vi "importAcq.vi"(7 "Probes":enum16{"Testing", "1-5", "6-10"}(ring)=enum."6-10", 8 "error in (no error)":errorcluster, 9 "Params":T1={"Mice ID"=[], "ExpType"=[], "Trial Interval"=[], "Pulse Duration"=[158.0, 152.0, 156.0, 167.0, 172.0], "microL_per_pulse"=[6.0, 6.0, 6.0, 6.0, 6.0], "Response Interval"=[1000.0, 1000.0, 1000.0, 1000.0, 1000.0], "Bad Delay"=[], "Response Period"=[], "liquid_type"="water", "Stimuli"=[], "Rewarded Stimuli"=[], "Air Dur"=50.0} {"Air Dur" format="%#_13g"}, 10 "REC":bool[](array[boolean]), 11 "Acquisition in":refnum<class "Acquisition.lvclass">) -> (0 "error out":errorcluster, 2 "# elements in queue":i32, 3 "Acquisition out":refnum<class "Acquisition.lvclass">)   [LabVIEW 2014, in "Acquisition.lvclass"]
uses:
  Acquisition.lvclass
  ParamsArray.ctl
  Acquisition.lvclass/Acquisition.ctl
  ParamsTuple.ctl
  Scanner/Database/Database.lvclass
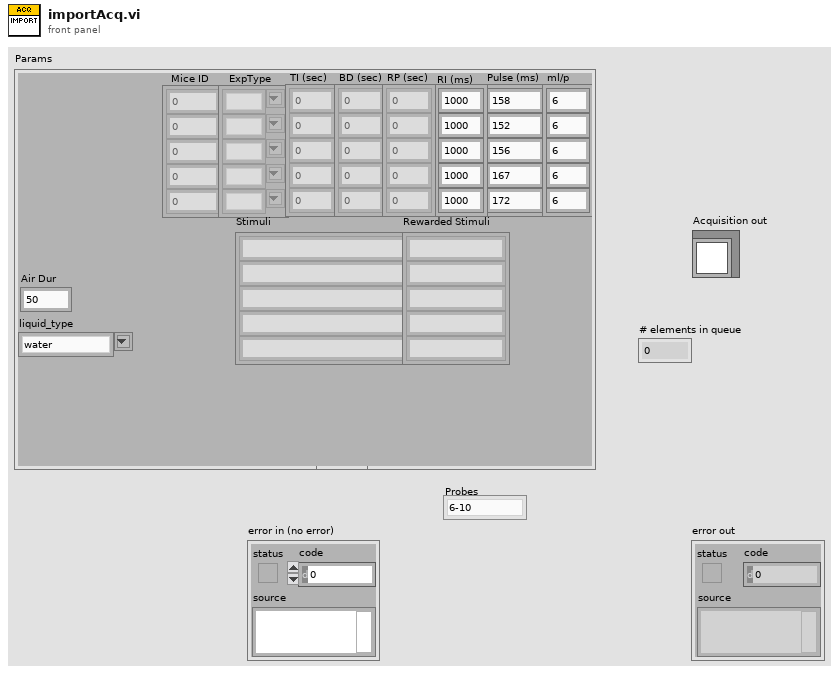
[diagram p1: front panel]
types:
  T1 = typedef "ParamsArray.ctl" = cluster{"Mice ID":dbl[], "ExpType":string[], "Trial Interval":dbl[], "Pulse Duration":dbl[], "microL_per_pulse":dbl[], "Response Interval":dbl[], "Bad Delay":dbl[], "Response Period":dbl[], "liquid_type":string, "Stimuli":string[], "Rewarded Stimuli":string[], "Air Dur":dbl}
  T2 = enum16{"air_delivery", "beh_session", "stim_periods", "licks", "liquid_delivery"}
  T3 = cluster{"mouse_id":dbl, "session_timestamp":string, "timestamp":dbl, "pulse_time":dbl, "microl_per_pulse":dbl, "liquid_type":string}
  T4 = cluster{"mouse_id":dbl, "session_timestamp":string, "timestamp":dbl, "pulse_time":dbl}
  T5 = cluster{"mouse_id":dbl, "session_timestamp":string, "timestamp":dbl}
  T6 = cluster{"mouse_id":dbl, "session_timestamp":string, "timestamp":dbl, "period_type":string}
  T7 = typedef "ParamsTuple.ctl" = cluster{"mouse_id":dbl, "session_timestamp":string, "trial_interval":dbl, "response_interval":dbl, "response_period":dbl, "bad_delay":dbl, "ExpType":string, "stimuli":string, "rewarded_stimuli":string, "setup":dbl}
  T8 = cluster{"table":enum16{"air_delivery", "beh_session", "stim_periods", "licks", "liquid_delivery"}, "timestamp":dbl, "Window Number (0...15)":i32, "period_type":string}
  T9 = typedef "ParamsArray2.ctl" = cluster{"liquid_type":string, "Mouse ID":dbl, "Trial Interval":dbl, "Pulse Duration":dbl, "microL_per_pulse":dbl, "Response Interval":dbl, "Bad Delay":dbl, "Response Period":dbl, "Stimuli":string, "Rewarded Stimuli":string, "Air Dur":dbl, "ExpType":string}
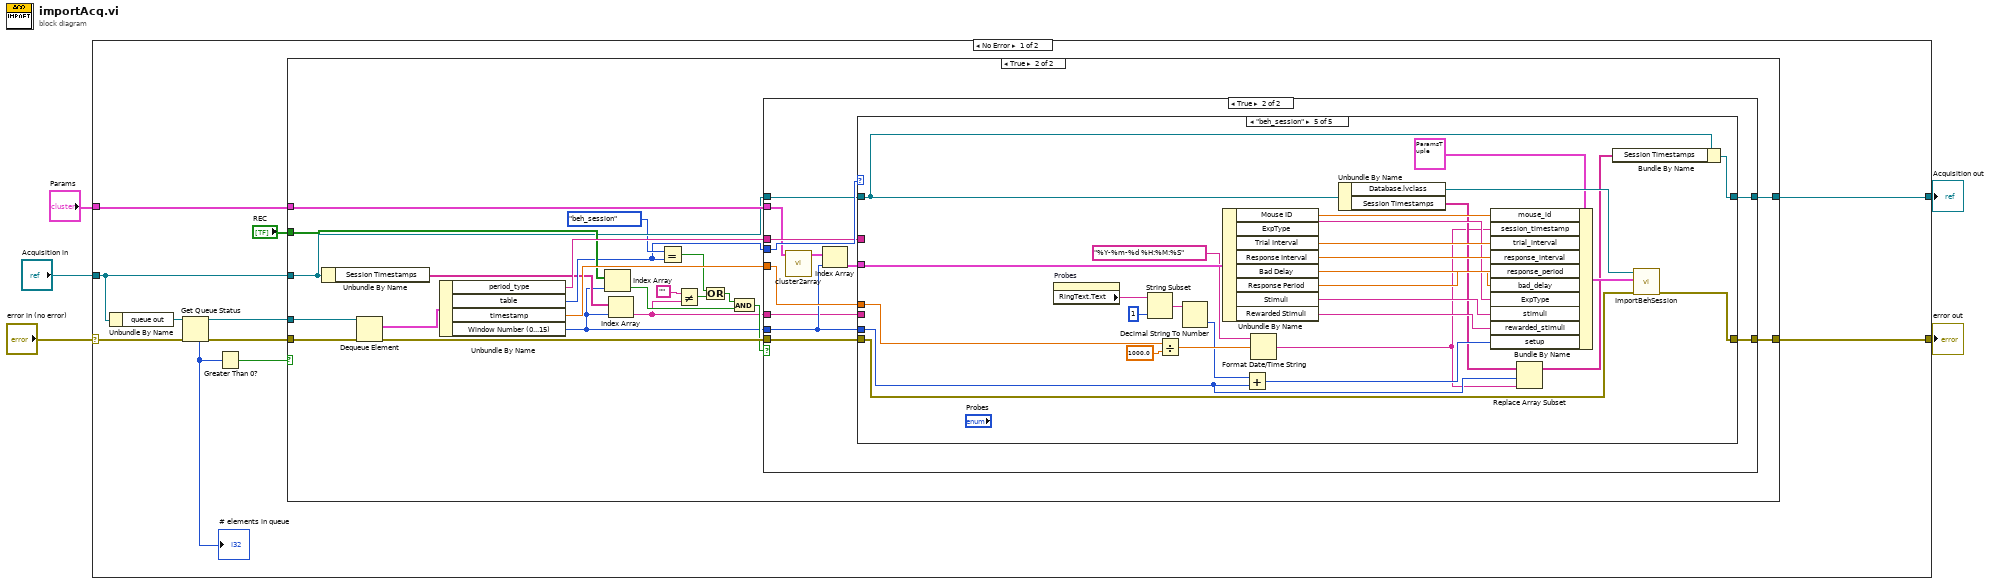
[diagram p0: block diagram]
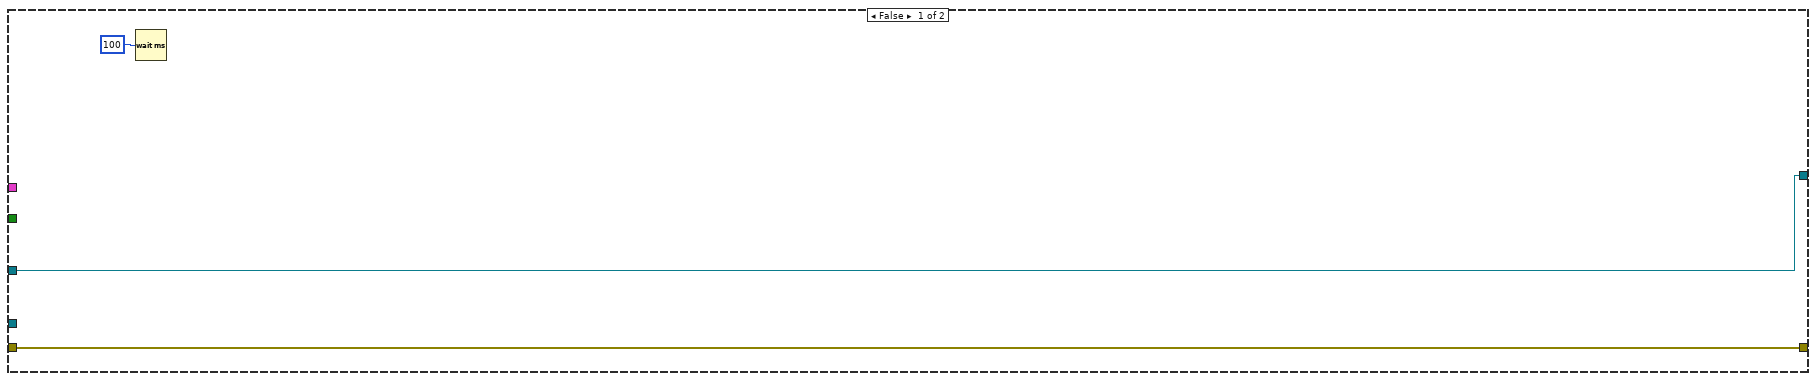
[diagram p2: hidden frame]
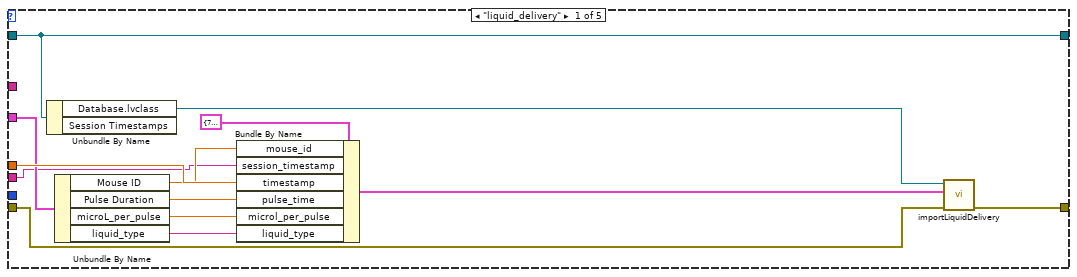
[diagram p4: hidden frame]
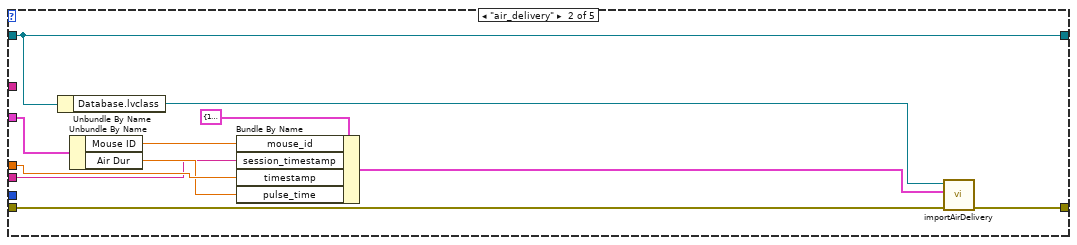
[diagram p5: hidden frame]
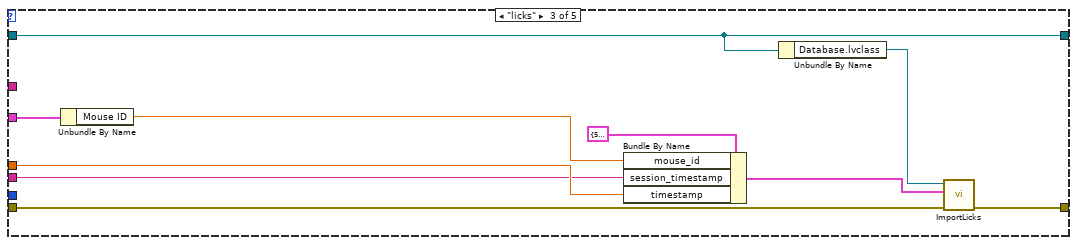
[diagram p6: hidden frame]
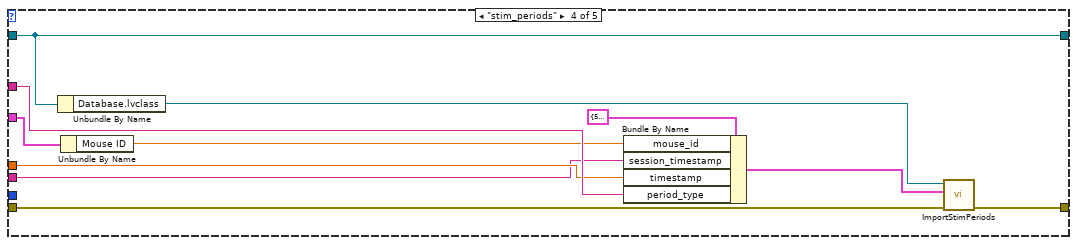
[diagram p7: hidden frame]
diagram:
  n1 = case shown="No Error" "error in (no error)" {
    selector: "error in (no error)" -> [w11 w131]
    tunnel: [w16 w131] -> w4
    tunnel: [w15 w130] -> w2
    tunnel: "Acquisition in" -> [w14 w130]
    tunnel: "Params" -> [w6 _]
    frame No Error {
      n2 = Unbundle By Name(w14) -> ("queue out"=w13:refnum<queue>)
      n3 = Get Queue Status(queue=w13, error in (no error)=w11) -> (queue out=w12:refnum<queue>, error out=w10:errorcluster, # elements in queue=w9:i32)  [unwired: 1 in, 5 out]
      "# elements in queue" <- w9
      n4 = Greater Than 0?(x=w9) -> (x > 0?=w8:bool)
      n5 = case shown="True" w8 {
        tunnel: [w18 w41] -> w16
        tunnel: w12 -> [_ w40]
        tunnel: [w17 w36] -> w15
        tunnel: w14 -> [w17 w31]
        tunnel: w10 -> [w18 w34]
        tunnel: "REC" -> [_ w33]
        tunnel: w6 -> [_ w32]
        frame False {
          n6 = Wait (ms)(milliseconds to wait=u32 100) -> ()  [unwired: 1 out]
        }
        frame True {
          n7 = Unbundle By Name(w31) -> ("Session Timestamps"=w22:string[])
          n8 = Dequeue Element(queue=w40, error in (no error)=w34) -> (element=w38:T8, error out=w39:errorcluster)  [unwired: 1 in, 2 out]
          n9 = Unbundle By Name(w38) -> ("period_type"=w35:string, "table"=w25:T2, "timestamp"=w37:dbl, "Window Number (0...15)"=w21:i32)
          n10 = Index Array(array=w33, index=w21) -> (element=w29:bool)
          n11 = Index Array(array=w22, index=w21) -> (element=w20:string)
          n12 = Equal?(x=T2."beh_session" ("table"), y=w25) -> (x = y?=w27:bool)
          n13 = Not Equal?(x="", y=w20) -> (x != y?=w24:bool)
          n14 = Or(x=w27, y=w24) -> (x .or. y?=w23:bool)
          n15 = And(x=w23, y=w29) -> (x .and. y?=w28:bool)
          n16 = case shown="True" w28 {
            tunnel: [w42 w55] -> w41
            tunnel: w39 -> [w42 w54]
            tunnel: w21 -> [_ w46]
            tunnel: w37 -> [_ w53]
            tunnel: [w43 w52] -> w36
            tunnel: w25 -> [_ w51]
            tunnel: w31 -> [w43 w50]
            tunnel: w35 -> [_ w49]
            tunnel: w32 -> [_ w48]
            tunnel: w20 -> [_ w44]
            frame False {
            }
            frame True {
              n17 = call "cluster2array.vi"("Params"=w48) -> ("Array"=w47:T9[])  [unwired: 10 in]
              n18 = Index Array(array=w47, index=w46) -> (element=w45:T9)
              n19 = case shown="\"beh_session\"" w51 {
                tunnel: w54 -> [w66 w76 w87 w97 w128]
                tunnel: [w65 w75 w86 w96 w127] -> w55
                tunnel: w46 -> [_ _ _ _ w103]
                tunnel: w53 -> [w63 w79 w84 w93 w114]
                tunnel: [w62 w78 w89 w95 w125] -> w52
                tunnel: w50 -> [w62 w78 w89 w95 w126]
                tunnel: w49 -> [_ _ _ w94 _]
                tunnel: w45 -> [w61 w72 w82 w92 w124]
                tunnel: w44 -> [w56 w69 w80 w90 _]
                frame "liquid_delivery" {
                  n20 = Unbundle By Name(w62) -> ("Database.lvclass"=w64:refnum<class "Database.lvclass">)  [unwired: 1 out]
                  n21 = Unbundle By Name(w61) -> ("Mouse ID"=w60:dbl, "Pulse Duration"=w59:dbl, "microL_per_pulse"=w58:dbl, "liquid_type"=w57:string)
                  n22 = Bundle By Name(cluster=T3 {"mouse_id"=76.0, "session_timestamp"="2015-04-13", "timestamp"=3511802490297.687, "pulse_time"=700.0, "microl_per_pulse"=12.0, "liquid_type"="water"} ("Tuple"), "mouse_id"=w60, "session_timestamp"=w56, "timestamp"=w63, "pulse_time"=w59, "microl_per_pulse"=w58, "liquid_type"=w57) -> (w67:T3)
                  n23 = call-dynamic "importLiquidDelivery.vi"("error in (no error)"=w66, "Tuple"=w67, "Database in"=w64) -> ("error out"=w65:errorcluster)  [unwired: 7 in, 1 out]
                }
                frame "air_delivery" {
                  n24 = Unbundle By Name(w78) -> ("Database.lvclass"=w77:refnum<class "Database.lvclass">)
                  n25 = Unbundle By Name(w72) -> ("Mouse ID"=w71:dbl, "Air Dur"=w70:dbl)
                  n26 = Bundle By Name(cluster=T4 {"mouse_id"=1217.0, "session_timestamp"="", "timestamp"=0.0, "pulse_time"=0.0} ("Tuple"), "mouse_id"=w71, "session_timestamp"=w69, "timestamp"=w79, "pulse_time"=w70) -> (w73:T4)
                  n27 = call-dynamic "importAirDelivery.vi"("error in (no error)"=w76, "Tuple"=w73, "Database in"=w77) -> ("error out"=w75:errorcluster)  [unwired: 7 in, 1 out]
                }
                frame "licks" {
                  n28 = Unbundle By Name(w82) -> ("Mouse ID"=w81:dbl)
                  n29 = Bundle By Name(cluster=T5 {"mouse_id"=5561.0, "session_timestamp"="2015-04-21", "timestamp"=3512495847309.028} ("Tuple"), "mouse_id"=w81, "session_timestamp"=w80, "timestamp"=w84) -> (w83:T5)
                  n30 = Unbundle By Name(w89) -> ("Database.lvclass"=w88:refnum<class "Database.lvclass">)
                  n31 = call-dynamic "ImportLicks.vi"("error in (no error)"=w87, "Tuple"=w83, "Database in"=w88) -> ("error out"=w86:errorcluster)  [unwired: 7 in, 1 out]
                }
                frame "stim_periods" {
                  n32 = Unbundle By Name(w95) -> ("Database.lvclass"=w100:refnum<class "Database.lvclass">)
                  n33 = Unbundle By Name(w92) -> ("Mouse ID"=w91:dbl)
                  n34 = Bundle By Name(cluster=T6 {"mouse_id"=5561.0, "session_timestamp"="2015-04-21", "timestamp"=3512495847309.028, "period_type"=""} ("Tuple"), "mouse_id"=w91, "session_timestamp"=w90, "timestamp"=w93, "period_type"=w94) -> (w98:T6)
                  n35 = call-dynamic "ImportStimPeriods.vi"("error in (no error)"=w97, "Tuple"=w98, "Database in"=w100) -> ("error out"=w96:errorcluster)  [unwired: 7 in, 1 out]
                }
                frame "beh_session" {
                  n36 = property on="Probes" class="Enum (strict)"() -> ("RingText.Text"=w108:string)  [unwired: 2 in, 2 out]
                  n37 = String Subset(string=w108, length (rest)=1 ("length (rest)")) -> (substring=w107:string)  [unwired: 1 in]
                  n38 = Divide(x=w114, y=1000.0) -> (x/y=w112:dbl)
                  n39 = Decimal String To Number(string=w107) -> (number=w106:i32)  [unwired: 2 in, 1 out]
                  n40 = Unbundle By Name(w124) -> ("Mouse ID"=w123:dbl, "ExpType"=w118:string, "Trial Interval"=w122:dbl, "Response Interval"=w121:dbl, "Bad Delay"=w119:dbl, "Response Period"=w120:dbl, "Stimuli"=w117:string, "Rewarded Stimuli"=w116:string)
                  n41 = Add(x=w106, y=w103) -> (x+y=w105:i32)
                  n42 = Format Date/Time String(time format string (%c)="%Y-%m-%d %H:%M:%S", seconds (now)=w112) -> (date/time string=w102:string)  [unwired: 1 in]
                  n43 = Unbundle By Name(w126) -> ("Database.lvclass"=w129:refnum<class "Database.lvclass">, "Session Timestamps"=w104:string[])
                  n44 = Bundle By Name(cluster=T7 {"mouse_id"=76.0, "session_timestamp"="2015-05-21 23-03-28", "trial_interval"=10.0, "response_interval"=1000.0, "response_period"=10.0, "bad_delay"=10.0, "ExpType"="Orientation", "stimuli"="0,90", "rewarded_stimuli"="0", "setup"=1.0} ("Tuple"), "mouse_id"=w123, "session_timestamp"=w102, "trial_interval"=w122, "response_interval"=w121, "response_period"=w120, "bad_delay"=w119, "ExpType"=w118, "stimuli"=w117, "rewarded_stimuli"=w116, "setup"=w105) -> (w111:T7)
                  n45 = Replace Array Subset(array=w104, new element=w102, index=w103) -> (w101:string[])
                  n46 = Bundle By Name(cluster=w126, "Session Timestamps"=w101) -> (w125:refnum<class "Acquisition.lvclass">)
                  n47 = call-dynamic "ImportBehSession.vi"("error in (no error)"=w128, "Tuple"=w111, "Database in"=w129) -> ("error out"=w127:errorcluster)  [unwired: 7 in, 1 out]
                }
              }
            }
          }
        }
      }
    }
    frame Error {
    }
  }
  "error out" <- w4
  "Acquisition out" <- w2
